vi "Data_Write.vi"(8 "Error In":errorcluster caption="错误输入", 10 "扫描参数":T1, 11 "数据文件对象":refnum<file>) -> (0 "Error Out":errorcluster caption="错误输出")   [LabVIEW 2020]
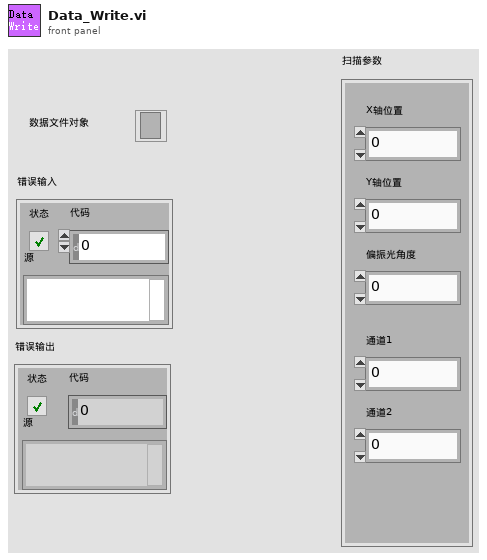
[diagram p1: front panel]
types:
  T1 = cluster{"X轴位置":dbl, "Y轴位置":dbl, "偏振光角度":dbl, "通道1":dbl, "通道2":dbl}
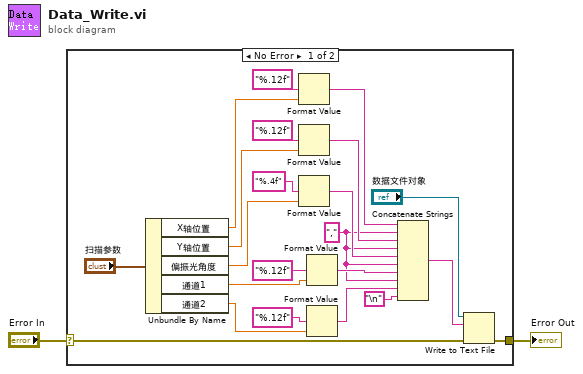
[diagram p0: block diagram]
diagram:
  n1 = case shown="No Error" "Error In" {
    selector: "Error In" -> [w23 w25]
    tunnel: [w22 w25] -> w1
    frame No Error {
      w4 = ","
      n2 = Unbundle By Name("扫描参数") -> ("X轴位置"=w19:dbl, "Y轴位置"=w20:dbl, "偏振光角度"=w21:dbl, "通道1"=w8:dbl, "通道2"=w7:dbl)
      n3 = Format Value(format string="%.12f", value (0)=w19) -> (output string=w15:string)  [unwired: 1 in]
      n4 = Format Value(format string="%.12f", value (0)=w20) -> (output string=w16:string)  [unwired: 1 in]
      n5 = Format Value(format string="%.4f", value (0)=w21) -> (output string=w17:string)  [unwired: 1 in]
      n6 = Format Value(format string="%.12f", value (0)=w8) -> (output string=w6:string)  [unwired: 1 in]
      n7 = Format Value(format string="%.12f", value (0)=w7) -> (output string=w5:string)  [unwired: 1 in]
      n8 = Concatenate Strings(w15, w4, w16, w4, w17, w4, w6, w4, w5, "\n") -> (w11:string)
      n9 = Write to Text File(file (use dialog)="数据文件对象", text=w11, error in=w23) -> (error out=w22:errorcluster)  [unwired: 1 in, 2 out]
    }
    frame Error {
    }
  }
  "Error Out" <- w1
